vi "SCU Test Main.vi"() -> ()   [LabVIEW 2014]
uses:
  Pressure Control/Pressure Control.lvclass
  TTL/TTL.lvclass
  Pressure Control/Pressure Control Config.ctl
panel:
  in  "DAQmx Device Name":tag="Dev3"
  in  "Laser Control 5":bool
  in  "Laser Control 4":bool
  in  "Laser Control 3":bool
  in  "Laser Control 2":bool
  in  "Laser Control 1":bool
  in  "Pressure Down":bool
  in  "Pressure Up":bool
  in  "Set zero pressure":bool caption="Vent pressure"
  in  "Vacuum":bool
  in  "Vent pressure":bool
  out "Pressure":dbl=-0.005982129914330336 format="%#.2f"
  in  "stop":bool
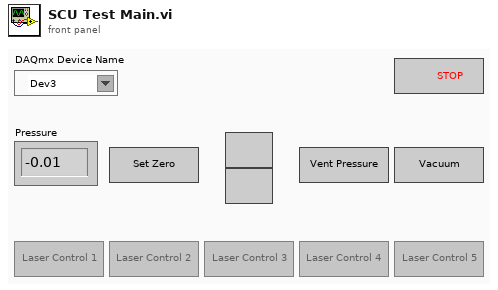
[diagram p1: front panel]
types:
  T1 = typedef "Pressure Control.lvclass/Pressure Control Config.ctl" = cluster{"daqmx_channel":string, "terminal_configuration":string}
  T2 = cluster{string, "TTL line # Pressure Up":u8, bool, bool}
  T3 = cluster{string, "TTL line # Pressure Down":u8, bool, bool}
  T4 = cluster{string, "TTL line # Pressure Vacuum":u8, bool, bool}
  T5 = cluster{string, "TTL line # Pressure Vacuum":u8, bool, bool}[]
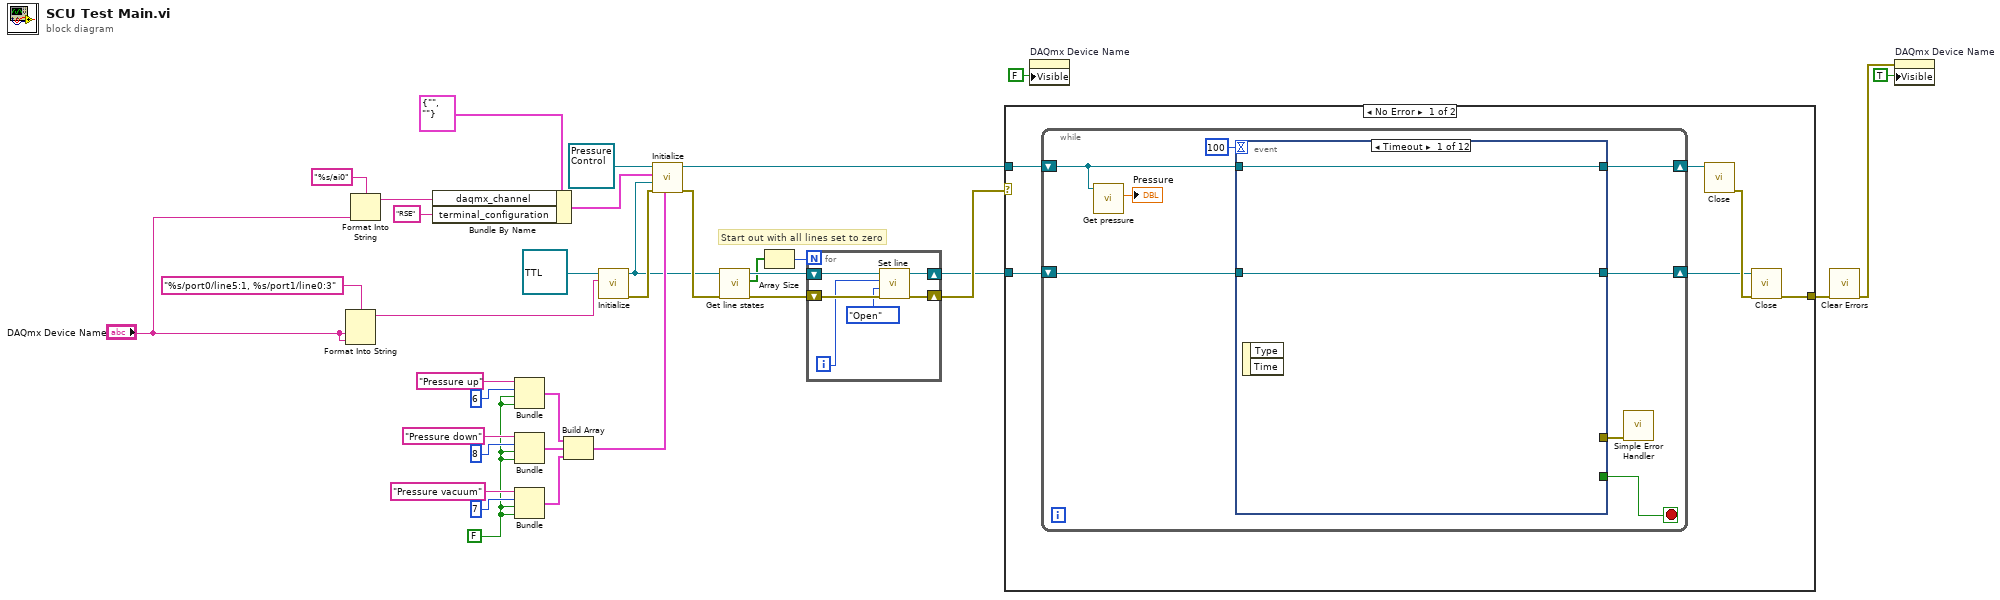
[diagram p0: block diagram]
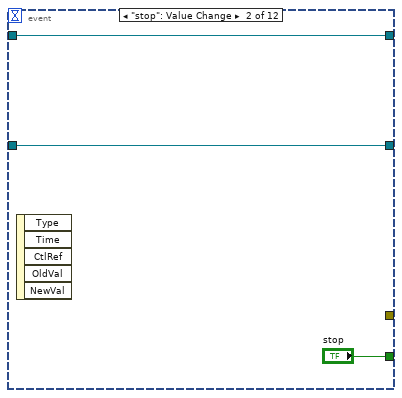
[diagram p2: hidden frame]
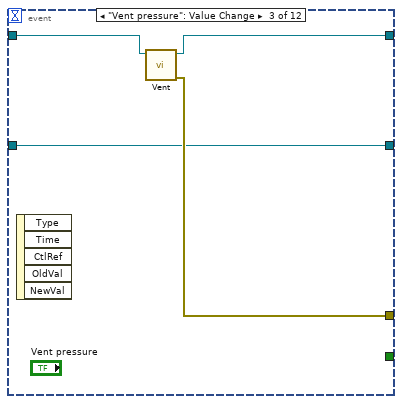
[diagram p3: hidden frame]
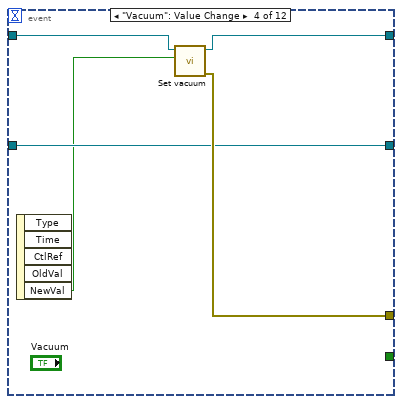
[diagram p4: hidden frame]
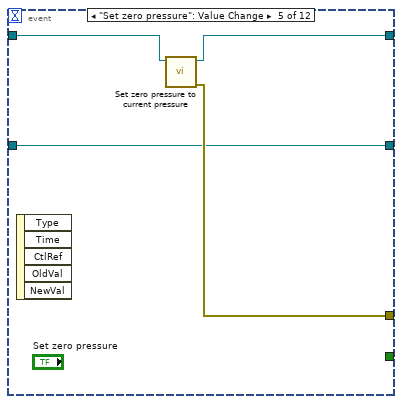
[diagram p5: hidden frame]
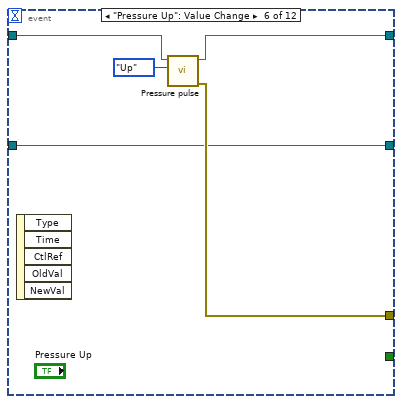
[diagram p6: hidden frame]
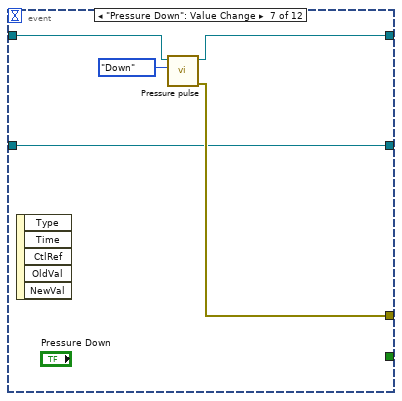
[diagram p7: hidden frame]
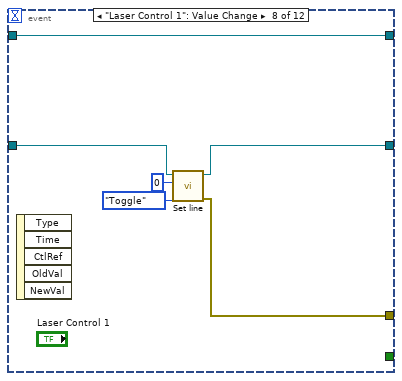
[diagram p8: hidden frame]
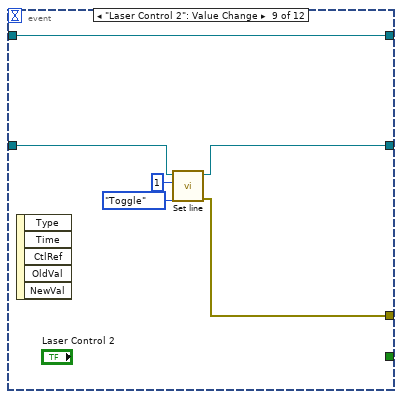
[diagram p9: hidden frame]
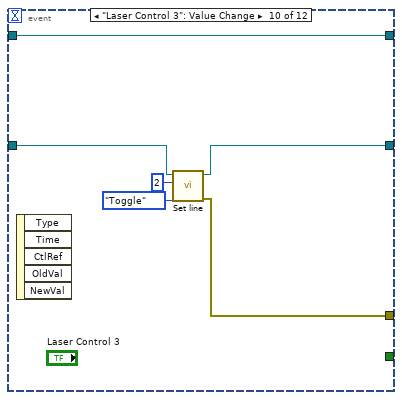
[diagram p10: hidden frame]
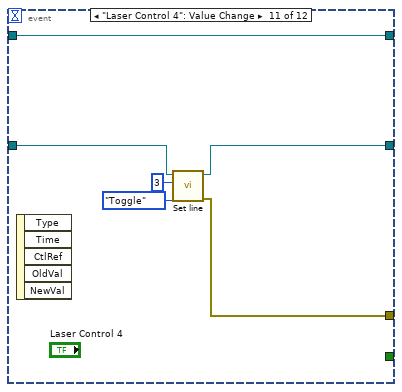
[diagram p11: hidden frame]
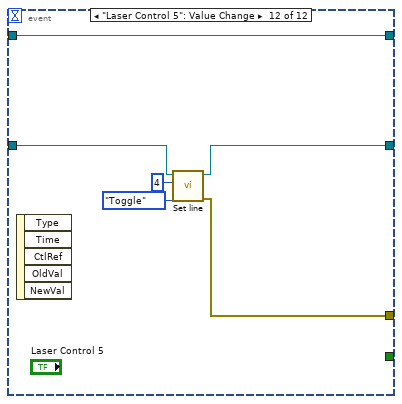
[diagram p12: hidden frame]
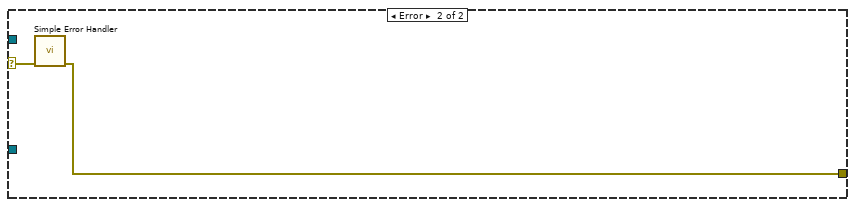
[diagram p13: hidden frame]
diagram:
  w22 = FALSE
  # "Start out with all lines set to zero"
  n1 = Format Into String(format string="%s/port0/line5:1, %s/port1/line0:3", "DAQmx Device Name", "DAQmx Device Name") -> (resulting string=w14:string)  [unwired: 2 in, 1 out]
  n2 = Format Into String(format string="%s/ai0", "DAQmx Device Name") -> (resulting string=w12:string)  [unwired: 2 in, 1 out]
  n3 = Bundle By Name(cluster=T1 {"daqmx_channel"="", "terminal_configuration"=""} ("Pressure Control Config"), "daqmx_channel"=w12, "terminal_configuration"="RSE") -> (w29:T1)
  n4 = Bundle("Pressure up", "TTL line # Pressure Up"=u8 6, w22, w22) -> (w20:T2)  [unwired: 1 in]
  n5 = Bundle("Pressure down", "TTL line # Pressure Down"=u8 8, w22, w22) -> (w21:T3)  [unwired: 1 in]
  n6 = Bundle("Pressure vacuum", "TTL line # Pressure Vacuum"=u8 7, w22, w22) -> (w19:T4)  [unwired: 1 in]
  n7 = Build Array(w20, w21, w19) -> (w18:T5)
  n8 = call "Initialize.vi"("TTL Ports"=w14, "TTL in"=refnum<class "TTL.lvclass"> refnum ("TTL.lvclass")) -> ("error out"=w17:errorcluster, "TTL out"=w6:refnum<class "TTL.lvclass">)  [unwired: 8 in]
  n9 = call "Initialize.vi"("TTL Lines"=w18, "error in (no error)"=w17, "TTL"=w6, "Pressure Control Config"=w29, "Pressure Control in"=refnum<class "Pressure Control.lvclass"> refnum ("Pressure Control.lvclass")) -> ("error out"=w34:errorcluster, "Pressure Control out"=w16:refnum<class "Pressure Control.lvclass">)  [unwired: 5 in]
  n10 = call "Get line states.vi"("error in (no error)"=w34, "TTL in"=w6) -> ("error out"=w1:errorcluster, "Current line states"=w2:bool[], "TTL out"=w5:refnum<class "TTL.lvclass">)  [unwired: 7 in]
  n11 = Array Size(array=w2) -> (size(s)=w3:i32)
  n12 = for {
    N: w3 -> [_]
    shift-right: [w40] -> w4
    shift-left: w5 -> [w41]
    shift-right: [w38] -> w35
    shift-left: w1 -> [w39]
    i -> [w37]
    n13 = call "Set line.vi"("error in (no error)"=w39, "Action"=enum16{"Open", "Close", "Toggle"}."Open", "Line number"=w37, "TTL in"=w41) -> ("error out"=w38:errorcluster, "TTL out"=w40:refnum<class "TTL.lvclass">)  [unwired: 6 in]
  }
  n14 = case shown="No Error" w35 {
    selector: w35 -> [_ w115]
    tunnel: w16 -> [w46 _]
    tunnel: w4 -> [w45 _]
    tunnel: [w42 w114] -> w9
    frame No Error {
      n15 = while {
        shift-right: [w54] -> w43
        shift-left: w46 -> [w53]
        shift-right: [w52] -> w44
        shift-left: w45 -> [w51]
        stop <- w49 stop-if-true
        n16 = call "Get pressure.vi"("Pressure Control in"=w53) -> ("Pressure"=→"Pressure":dbl)  [unwired: 7 in, 3 out]
        n17 = event shown="[0] Timeout" {
          selector: _ -> [_ _ _ _ _ _ _ _ _ _ _ _]
          dyn-events: _ -> [_ _ _ _ _ _ _ _ _ _ _ _]
          timeout: 100 -> [_ _ _ _ _ _ _ _ _ _ _ _]
          tunnel: [w57 w59 w61 w66 w70 w75 w80 w89 w95 w101 w107 w113] -> w54
          tunnel: w53 -> [w57 w59 w62 w67 w71 w76 w81 w89 w95 w101 w107 w113]
          tunnel: [w56 w58 w63 w68 w72 w77 w82 w87 w93 w99 w105 w111] -> w52
          tunnel: w51 -> [w56 w58 w63 w68 w72 w77 w82 w88 w94 w100 w106 w112]
          tunnel: [_ "stop" _ _ _ _ _ _ _ _ _ _] -> w49
          tunnel: [_ _ w64 w69 w73 w78 w83 w84 w90 w96 w102 w108] -> w48
          event Timeout {
            n18 = event-data() -> ()  [unwired: 1 in, 2 out]
          }
          event "stop": Value Change {
            n19 = event-data() -> ()  [unwired: 1 in, 5 out]
          }
          event "Vent pressure": Value Change {
            n20 = event-data() -> ()  [unwired: 1 in, 5 out]
            n21 = call "Vent.vi"("Pressure Control in"=w62) -> ("error out"=w64:errorcluster, "Pressure Control out"=w61:refnum<class "Pressure Control.lvclass">)  [unwired: 9 in]
          }
          event "Vacuum": Value Change {
            n22 = event-data() -> ("NewVal"=w65:bool)  [unwired: 1 in, 4 out]
            n23 = call "Set vacuum.vi"("Vacuum?"=w65, "Pressure Control in"=w67) -> ("error out"=w69:errorcluster, "Pressure Control out"=w66:refnum<class "Pressure Control.lvclass">)  [unwired: 8 in]
          }
          event "Set zero pressure": Value Change {
            n24 = event-data() -> ()  [unwired: 1 in, 5 out]
            n25 = call "Set zero pressure to current pressure.vi"("Pressure Control in"=w71) -> ("error out"=w73:errorcluster, "Pressure Control out"=w70:refnum<class "Pressure Control.lvclass">)  [unwired: 8 in, 1 out]
          }
          event "Pressure Up": Value Change {
            n26 = event-data() -> ()  [unwired: 1 in, 5 out]
            n27 = call "Pressure pulse.vi"("Up or down?"=enum16{"Up", "Down"}."Up", "Pressure Control in"=w76) -> ("error out"=w78:errorcluster, "Pressure Control out"=w75:refnum<class "Pressure Control.lvclass">)  [unwired: 8 in]
          }
          event "Pressure Down": Value Change {
            n28 = event-data() -> ()  [unwired: 1 in, 5 out]
            n29 = call "Pressure pulse.vi"("Up or down?"=enum16{"Up", "Down"}."Down", "Pressure Control in"=w81) -> ("error out"=w83:errorcluster, "Pressure Control out"=w80:refnum<class "Pressure Control.lvclass">)  [unwired: 8 in]
          }
          event "Laser Control 1": Value Change {
            n30 = event-data() -> ()  [unwired: 1 in, 5 out]
            n31 = call "Set line.vi"("Action"=enum16{"Open", "Close", "Toggle"}."Toggle", "Line number"=u8 0, "TTL in"=w88) -> ("error out"=w84:errorcluster, "TTL out"=w87:refnum<class "TTL.lvclass">)  [unwired: 7 in]
          }
          event "Laser Control 2": Value Change {
            n32 = event-data() -> ()  [unwired: 1 in, 5 out]
            n33 = call "Set line.vi"("Action"=enum16{"Open", "Close", "Toggle"}."Toggle", "Line number"=u8 1, "TTL in"=w94) -> ("error out"=w90:errorcluster, "TTL out"=w93:refnum<class "TTL.lvclass">)  [unwired: 7 in]
          }
          event "Laser Control 3": Value Change {
            n34 = event-data() -> ()  [unwired: 1 in, 5 out]
            n35 = call "Set line.vi"("Action"=enum16{"Open", "Close", "Toggle"}."Toggle", "Line number"=u8 2, "TTL in"=w100) -> ("error out"=w96:errorcluster, "TTL out"=w99:refnum<class "TTL.lvclass">)  [unwired: 7 in]
          }
          event "Laser Control 4": Value Change {
            n36 = event-data() -> ()  [unwired: 1 in, 5 out]
            n37 = call "Set line.vi"("Action"=enum16{"Open", "Close", "Toggle"}."Toggle", "Line number"=u8 3, "TTL in"=w106) -> ("error out"=w102:errorcluster, "TTL out"=w105:refnum<class "TTL.lvclass">)  [unwired: 7 in]
          }
          event "Laser Control 5": Value Change {
            n38 = event-data() -> ()  [unwired: 1 in, 5 out]
            n39 = call "Set line.vi"("Action"=enum16{"Open", "Close", "Toggle"}."Toggle", "Line number"=u8 4, "TTL in"=w112) -> ("error out"=w108:errorcluster, "TTL out"=w111:refnum<class "TTL.lvclass">)  [unwired: 7 in]
          }
        }
        n40 = call <vilib>:"Simple Error Handler.vi"("error in (no error)"=w48) -> ()  [unwired: 4 in, 5 out]
      }
      n41 = call "Close.vi"("Pressure Control in"=w43) -> ("error out"=w47:errorcluster)  [unwired: 9 in, 1 out]
      n42 = call "Close.vi"("error in (no error)"=w47, "TTL in"=w44) -> ("error out"=w42:errorcluster)  [unwired: 8 in, 1 out]
    }
    frame Error {
      n43 = call <vilib>:"Simple Error Handler.vi"("error in (no error)"=w115) -> ("error out"=w114:errorcluster)  [unwired: 4 in, 4 out]
    }
  }
  n44 = property on="DAQmx Device Name" class="DAQmxName"("Visible"=FALSE) -> ()  [unwired: 2 in, 2 out]
  n45 = call <vilib>:"Clear Errors.vi"("error in (no error)"=w9) -> ("error out"=w7:errorcluster)  [unwired: 5 in, 1 out]
  n46 = property on="DAQmx Device Name" class="DAQmxName"(error in=w7, "Visible"=TRUE) -> ()  [unwired: 1 in, 2 out]
